vi "copyright PC.vi"() -> ()   [LabVIEW 2010]
uses:
  ADT 2/help.ctl
panel:
  in  "OK Button":bool
  in  "Help Button":T1
  # "Process Controller 2.0\nData Acquisition and Control"
  # "©2004 Cornell University\nall rights reserved\n\nAuthored by Monroe Weber-Shirk\nmw24@cornell.edu\n\nDocumentation available at:\nwww.cee.cornell.edu/mw24/software\nCivil and Environmental Engineering\nCornell University"
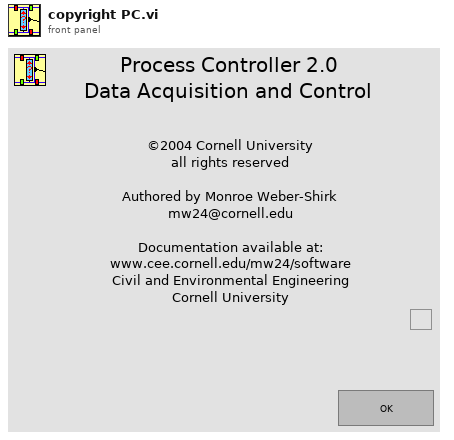
[diagram p1: front panel]
types:
  T1 = typedef "help.ctl" = bool
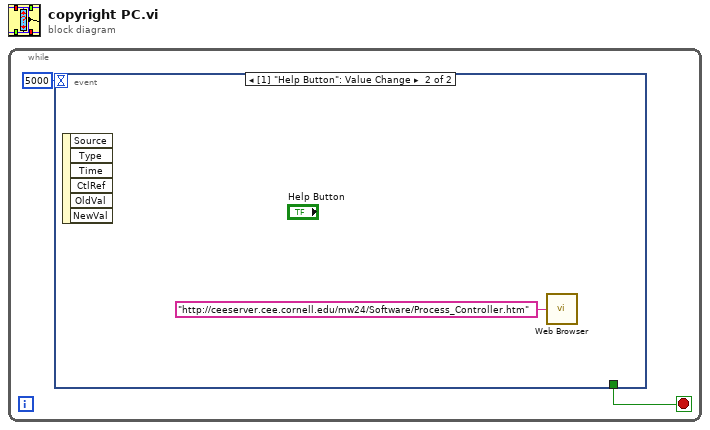
[diagram p0: block diagram]
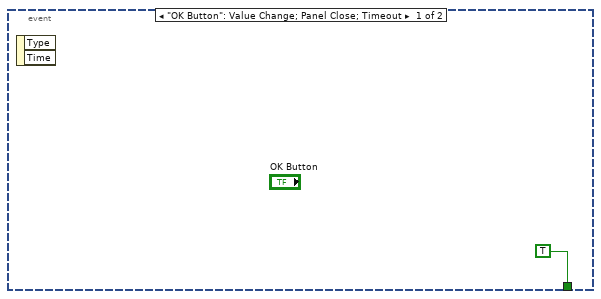
[diagram p2: hidden frame]
diagram:
  n1 = while {
    stop <- w2 stop-if-true
    n2 = event shown="[1] \"Help Button\": Value Change" {
      selector: _ -> [_ _]
      dyn-events: _ -> [_ _]
      timeout: 5000 -> [_ _]
      tunnel: [TRUE _] -> w2
      event "OK Button": Value Change; Panel Close; Timeout {
        n3 = event-data() -> ()  [unwired: 1 in, 2 out]
      }
      event Value Change {
        n4 = event-data() -> ()  [unwired: 1 in, 6 out]
        n5 = call "Web Browser.vi"("URL"="http://ceeserver.cee.cornell.edu/mw24/Software/Process_Controller.htm") -> ()  [unwired: 1 in]
      }
    }
  }
